vi "MVE Network Browse.vi"(10 "Item Path":string, 11 "in path":string) -> (3 "out path":string)   [LabVIEW 2016]
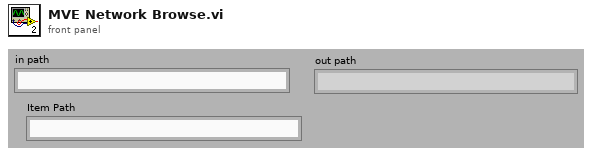
[diagram p1: front panel]
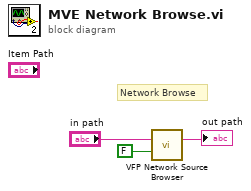
[diagram p0: block diagram]
diagram:
  # "Network Browse"
  n1 = call <resource>:"VFP Network Source Browser.vi"("InitPath"="in path", "MatchChkBox(T)?"=FALSE) -> ("outPath"=→"out path":string)  [unwired: 8 in, 5 out]
